vi "Read Serial Input Channel Status.vi"(0 "fpga interface in":refnum<k20>, 11 "error in (no error)":errorcluster) -> (4 "fpga interface out":refnum<k20>, 6 "serial input channel status":T1(array[cluster])=[{"acq state"=enum."Idle", "stop timed out"=FALSE, "bad packet header"=FALSE, "bad packet payload"=FALSE, "bad packet size"=FALSE, "dram status"={"bytes written"=0, "bytes read"=0, "overflow"=FALSE, "partition full"=FALSE, "last byte flushed"=FALSE}}, {"acq state"=enum."Idle", "stop timed out"=FALSE, "bad packet header"=FALSE, "bad packet payload"=FALSE, "bad packet size"=FALSE, "dram status"={"bytes written"=0, "bytes read"=0, "overflow"=FALSE, "partition full"=FALSE, "last byte flushed"=FALSE}}, {"acq state"=enum."Idle", "stop timed out"=FALSE, "bad packet header"=FALSE, "bad packet payload"=FALSE, "bad packet size"=FALSE, "dram status"={"bytes written"=0, "bytes read"=0, "overflow"=FALSE, "partition full"=FALSE, "last byte flushed"=FALSE}}, {"acq state"=enum."Idle", "stop timed out"=FALSE, "bad packet header"=FALSE, "bad packet payload"=FALSE, "bad packet size"=FALSE, "dram status"={"bytes written"=0, "bytes read"=0, "overflow"=FALSE, "partition full"=FALSE, "last byte flushed"=FALSE}}, {"acq state"=enum."Idle", "stop timed out"=FALSE, "bad packet header"=FALSE, "bad packet payload"=FALSE, "bad packet size"=FALSE, "dram status"={"bytes written"=0, "bytes read"=0, "overflow"=FALSE, "partition full"=FALSE, "last byte flushed"=FALSE}}, {"acq state"=enum."Idle", "stop timed out"=FALSE, "bad packet header"=FALSE, "bad packet payload"=FALSE, "bad packet size"=FALSE, "dram status"={"bytes written"=0, "bytes read"=0, "overflow"=FALSE, "partition full"=FALSE, "last byte flushed"=FALSE}}, {"acq state"=enum."Idle", "stop timed out"=FALSE, "bad packet header"=FALSE, "bad packet payload"=FALSE, "bad packet size"=FALSE, "dram status"={"bytes written"=0, "bytes read"=0, "overflow"=FALSE, "partition full"=FALSE, "last byte flushed"=FALSE}}, {"acq state"=enum."Idle", "stop timed out"=FALSE, "bad packet header"=FALSE, "bad packet payload"=FALSE, "bad packet size"=FALSE, "dram status"={"bytes written"=0, "bytes read"=0, "overflow"=FALSE, "partition full"=FALSE, "last byte flushed"=FALSE}}], 15 "error out":errorcluster)   [LabVIEW 2023, in "GettingStarted_Common_148X_Host.lvlib"]
uses:
  GettingStarted_Common_148X_Host.lvlib
  Acq/Types/148x_Acq_FPGA_Reference.ctl
  <vilib>/Utility/error.llb/Error Cluster From Error Code.vi
  <vilib>/rvi/errors/niLvFpgaAdjustHostInterfaceError.vi
  <vilib>/rvi/interface/nirviReadWriteControl/nirviReadWriteControl.xnode
  Acq/GettingStarted_Acq_148X_Host.lvlib
  NiFpgaLv.dll
  <vilib>/rvi/interface/Simulation/niFpgaSimulationCallBeginRW.vi
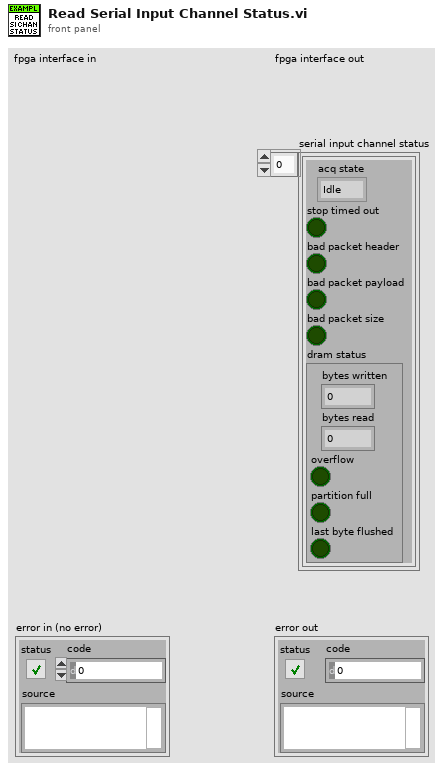
[diagram p1: front panel]
types:
  T1 = cluster{"acq state":enum8{"Idle", "Wait for First Packet Header", "Acquire", "Wait for Last Packet Header", "Wait for End of Last Packet"}, "stop timed out":bool, "bad packet header":bool, "bad packet payload":bool, "bad packet size":bool, "dram status":cluster{"bytes written":u64, "bytes read":u64, "overflow":bool, "partition full":bool, "last byte flushed":bool}}[]
  T2 = typedef "GettingStarted_Acq_148X_Host.lvlib/148x_Acq_FPGA_Reference.ctl" = refnum<k20>
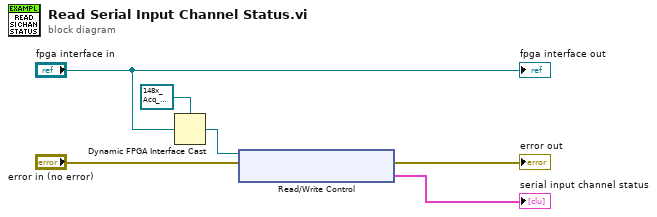
[diagram p0: block diagram]
diagram:
  n1 = Dynamic FPGA Interface Cast(Session In=T2 refnum ("FPGA VI Reference Out"), Type="fpga interface in") -> (Session Out=w6:T2)
  n2 = xnode "Read/Write Control"("FPGA VI Reference In"=w6, "error in"="error in (no error)") -> ("error out"=→"error out":errorcluster, "serial input channel status"=→"serial input channel status":T1)  [unwired: 1 out]
  "fpga interface out" <- "fpga interface in"
